vi "MultipleMeasurements.vi"(8 "error in (no error)":errorcluster, 10 "Time in ms (30000)":u32=30000, 11 "VISA resource name":refnum<visa-resource-name>) -> (0 "error out":errorcluster, 1 "Raw output":dbl[](array[numeric]), 2 "output/s":dbl[](array[numeric]), 3 "VISA resource name out":refnum<visa-resource-name>)   [LabVIEW 2014, in "GP22_TDC_Arduinoed.lvlib"]
doc: "Measure the time between triggers and output an array of all these measurements in the given measurement period."
uses:
  GP22_TDC_Arduinoed.lvlib
  Private/ConvertTimes - Array.vi
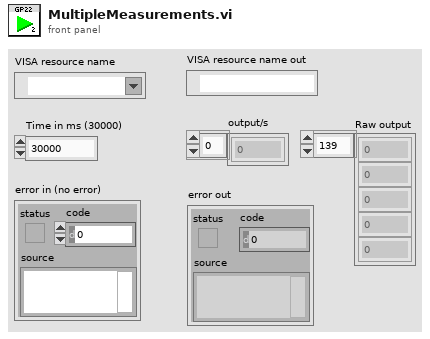
[diagram p1: front panel]
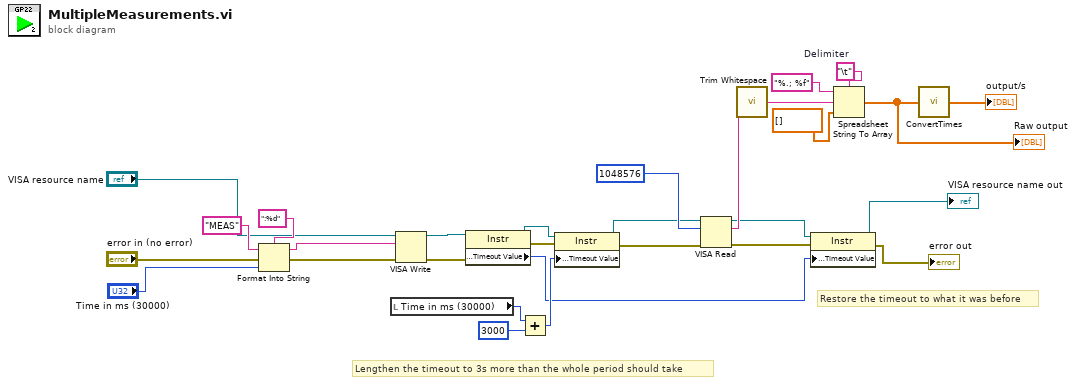
[diagram p0: block diagram]
diagram:
  w21 = "\t"  # Delimiter
  # "Restore the timeout to what it was before"
  # "Lengthen the timeout to 3s more than the whole period should take"
  n1 = Format Into String(format string=":%d", initial string="MEAS" ("command"), error in="error in (no error)", "Time in ms (30000)") -> (resulting string=w23:string, error out=w27:errorcluster)
  n2 = local read "Time in ms (30000)"() -> (w10:u32)
  n3 = VISA Write(VISA resource name="VISA resource name", write buffer=w23, error in (no error)=w27) -> (VISA resource name out=w17:refnum<visa-resource-name>, error out=w16:errorcluster)  [unwired: 1 out]
  n4 = property class="Instr"(reference=w17, error in=w16) -> (reference out=w15:refnum<visa-resource-name>, error out=w14:errorcluster, "General Settings:Timeout Value"=w4:u32)
  n5 = Add(x=w10, y=3000) -> (x+y=w11:u32)
  n6 = property class="Instr"(reference=w15, error in=w14, "General Settings:Timeout Value"=w11) -> (reference out=w13:refnum<visa-resource-name>, error out=w12:errorcluster)
  n7 = VISA Read(VISA resource name=w13, byte count=u32 1048576, error in (no error)=w12) -> (VISA resource name out=w8:refnum<visa-resource-name>, read buffer=w18:string, error out=w7:errorcluster)  [unwired: 1 out]
  n8 = call <vilib>:"Trim Whitespace.vi"("string"=w18) -> ("trimmed string"=w1:string)  [unwired: 1 in]
  n9 = property class="Instr"(reference=w8, error in=w7, "General Settings:Timeout Value"=w4) -> (reference out=→"VISA resource name out":refnum<visa-resource-name>, error out=→"error out":errorcluster)
  n10 = Spreadsheet String To Array(delimiter (Tab)=w21, format string="%.; %f", spreadsheet string=w1, array type (2D Dbl)=dbl[] []) -> (array=w2:dbl[])
  "Raw output" <- w2
  n11 = call-poly "ConvertTimes.vi"("GP22 results"=w2) -> ("Array of times / s"=→"output/s":dbl[])
